vi "RT VI.vi"() -> ()   [LabVIEW 2014]
uses:
  Timer 2013/Control Timer.ctl
  <vilib>/ptbypt/NI_PtbyPt.lvlib
panel:
  out "SDFlag":bool
  in  "Emergency off":bool
  in  "Right":bool
  in  "Center":bool
  in  "Left":bool
  in  "Off":bool
  in  "On":bool
  out "On/Off":bool
  out "BrojacGreska":dbl
  out "Brojac":dbl
  out "Fault":bool
  out "RightLED":bool
  out "CenterLED":bool
  out "LeftLED":bool
  out "Stanje":string
  out "error out":errorcluster
  in  "error in (no error)":errorcluster
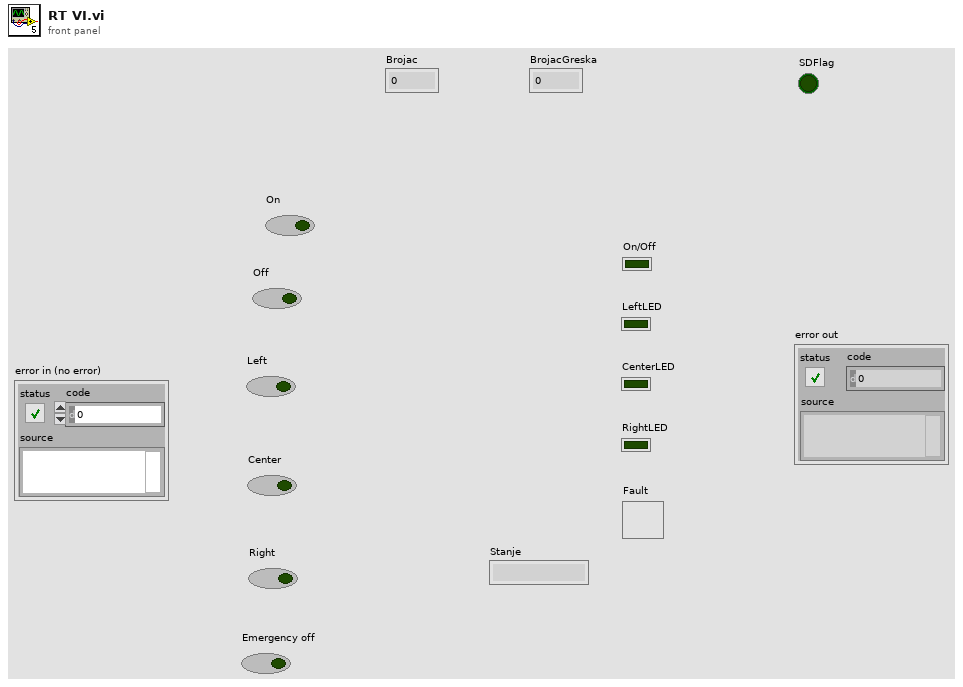
[diagram p1: front panel]
types:
  T1 = typedef "Control Timer.ctl" = enum16{"Timecheck", "Reset"}
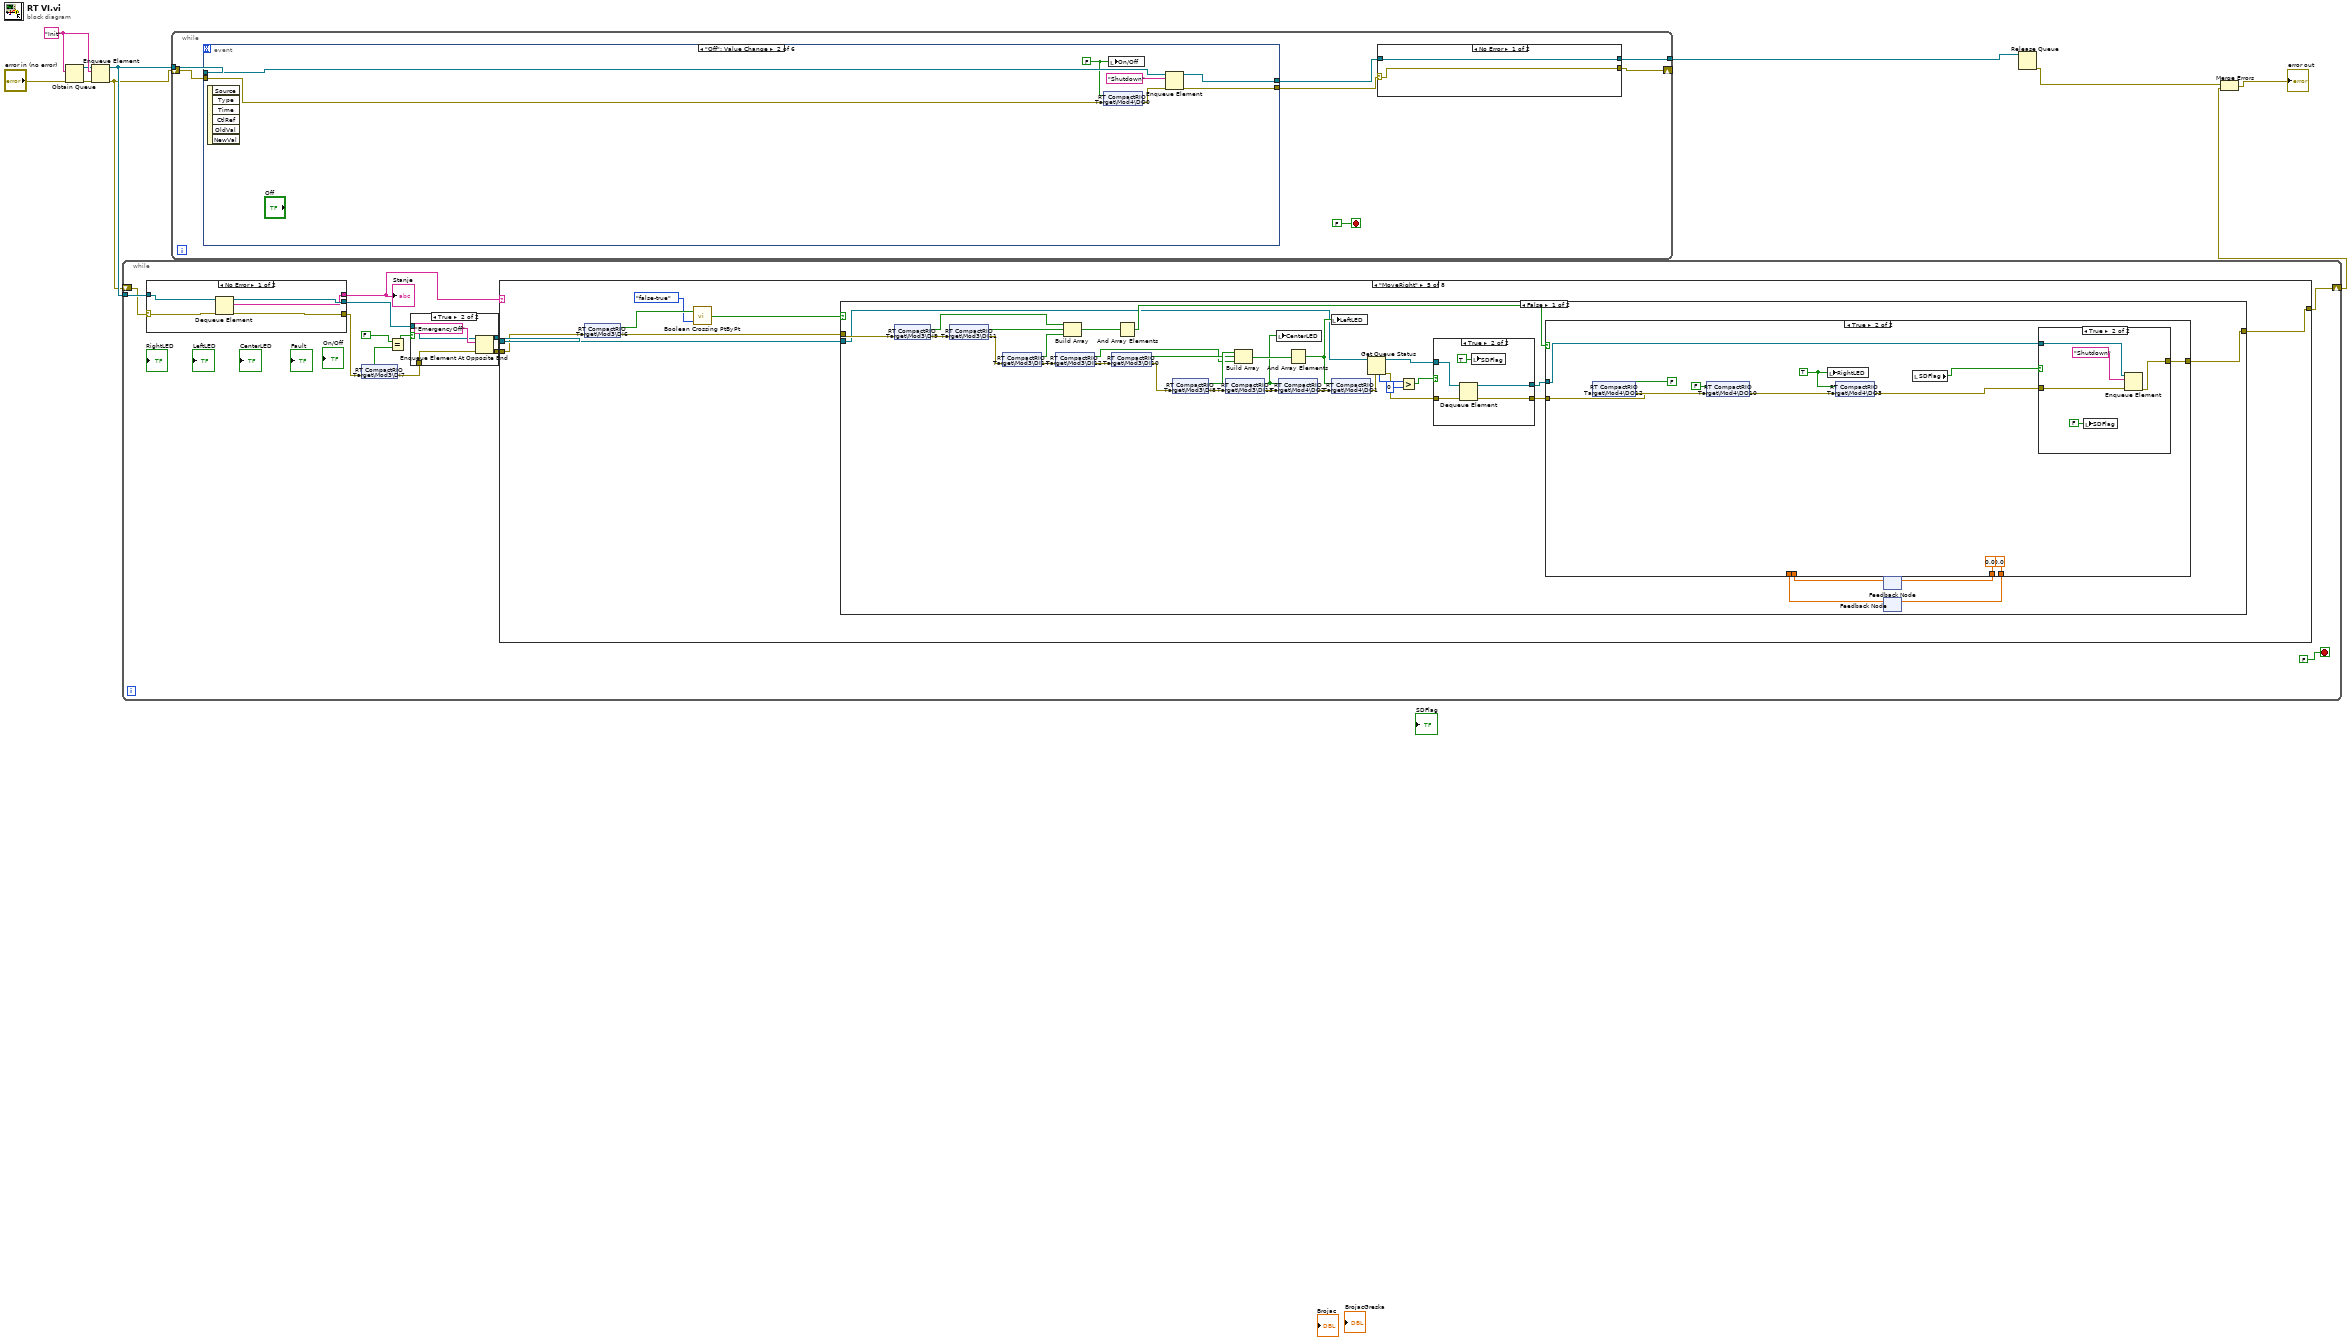
[diagram p0: block diagram]
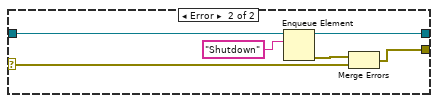
[diagram p2: hidden frame]
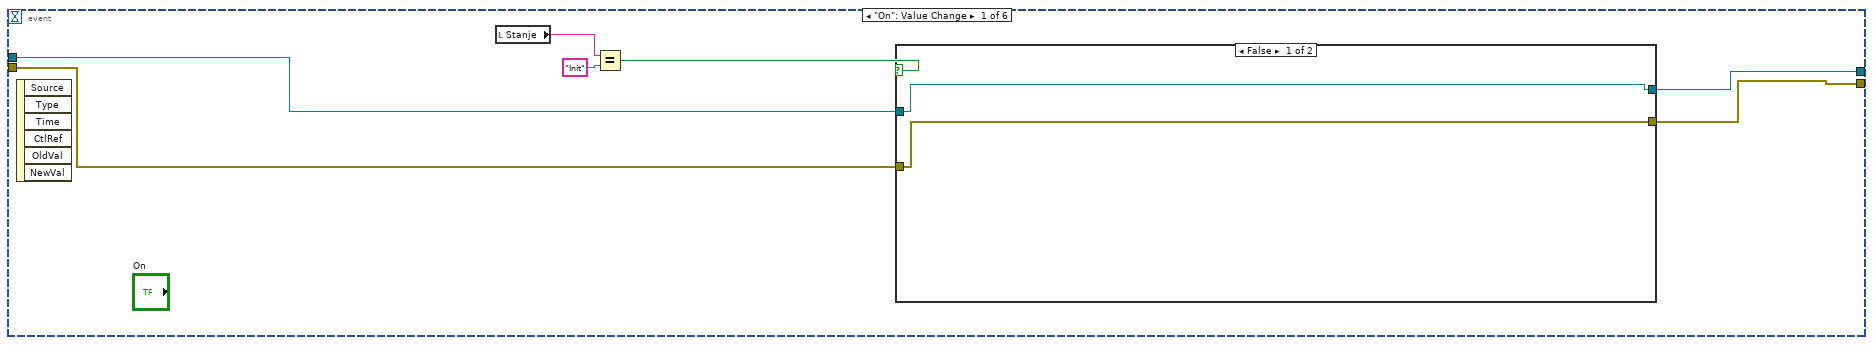
[diagram p3: hidden frame]
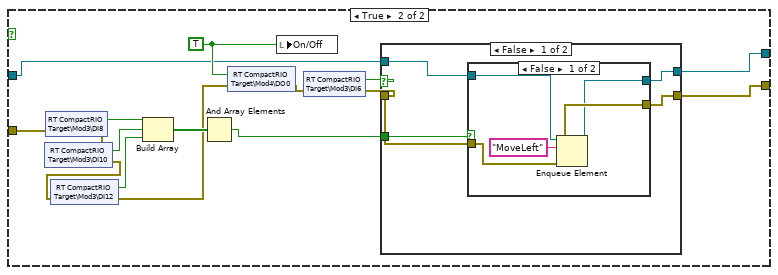
[diagram p4: hidden frame]
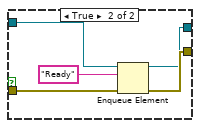
[diagram p5: hidden frame]
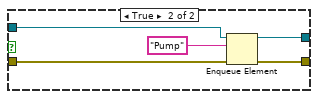
[diagram p6: hidden frame]
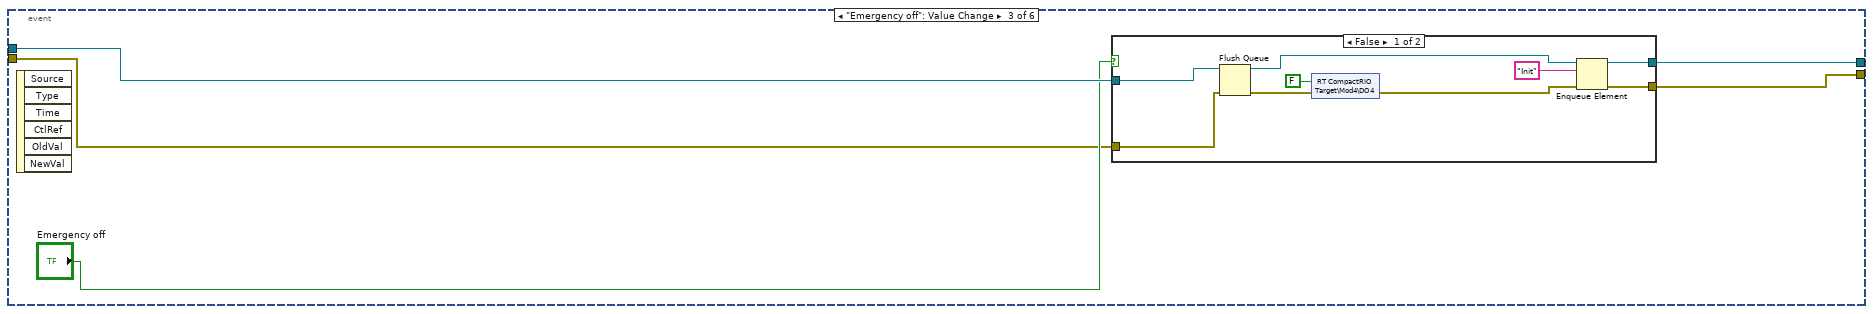
[diagram p7: hidden frame]
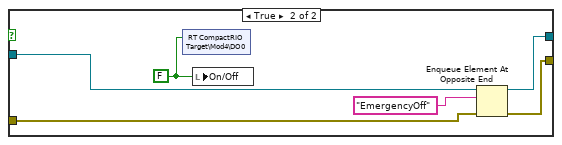
[diagram p8: hidden frame]
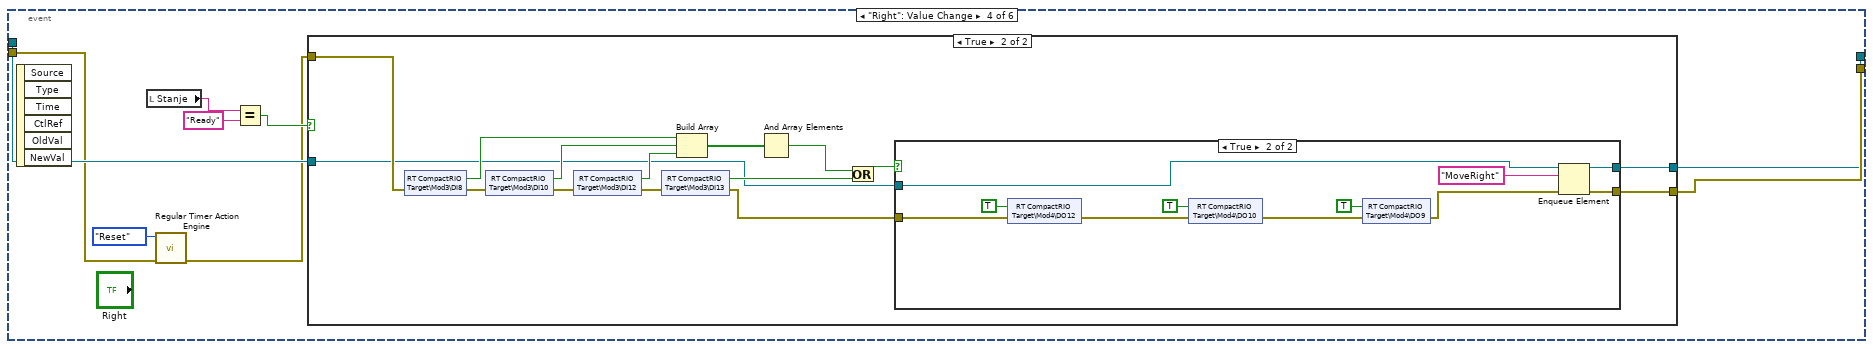
[diagram p9: hidden frame]
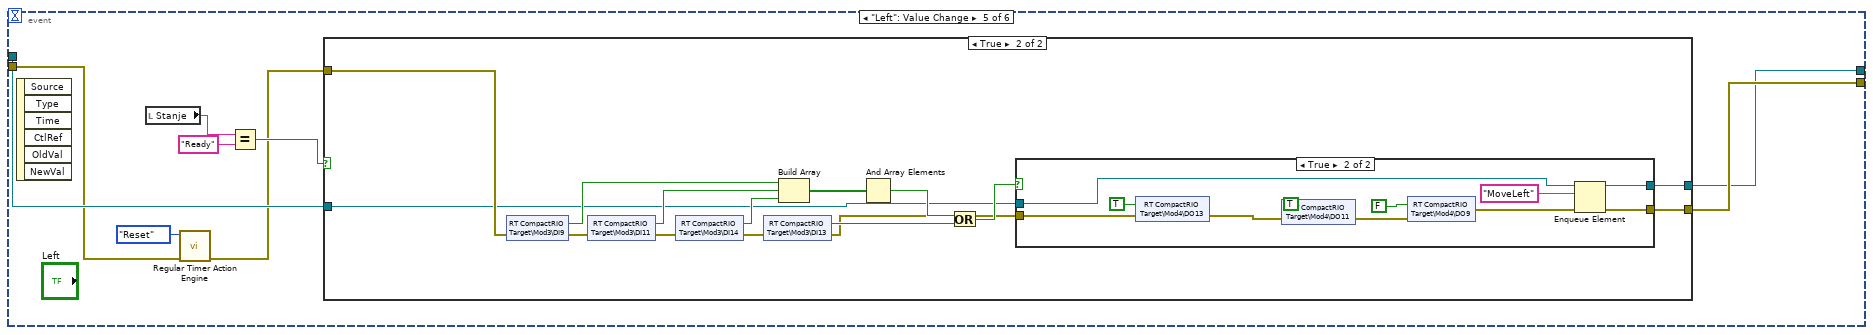
[diagram p12: hidden frame]
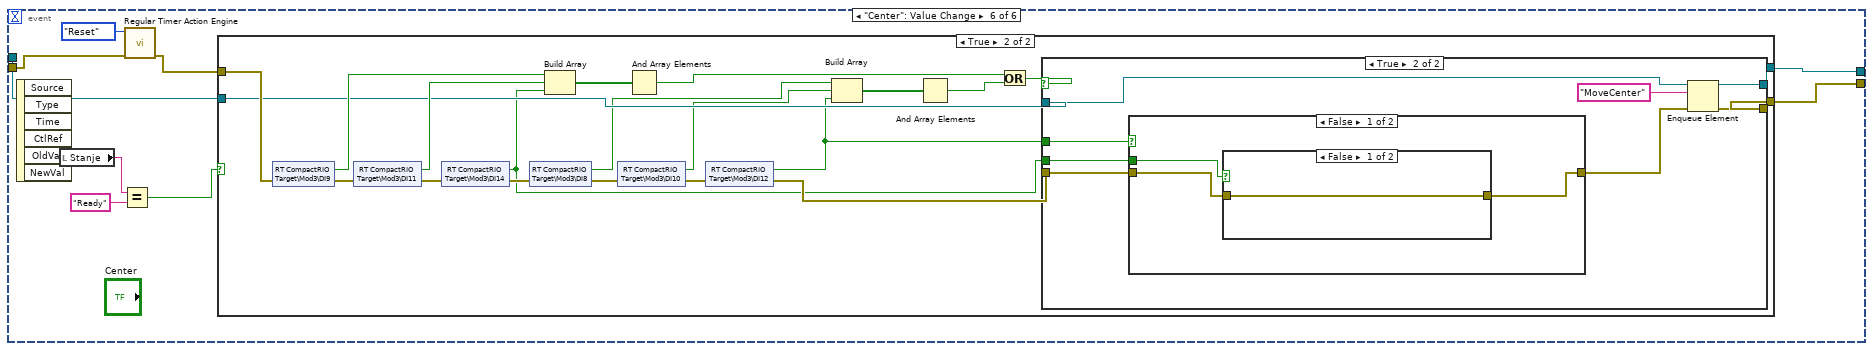
[diagram p15: hidden frame]
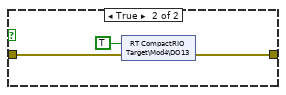
[diagram p18: hidden frame]
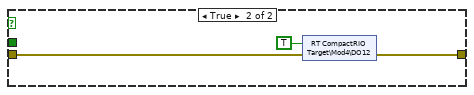
[diagram p19: hidden frame]
diagram:
  w10 = "Init"
  n1 = Obtain Queue(element data type=w10, error in (no error)="error in (no error)") -> (queue out=w8:refnum<queue>, error out=w9:errorcluster)  [unwired: 3 in, 1 out]
  n2 = Enqueue Element(queue=w8, element=w10, error in (no error)=w9) -> (queue out=w7:refnum<queue>, error out=w2:errorcluster)  [unwired: 1 in, 1 out]
  n3 = while {
    tunnel: w7 -> [w23]
    shift-right: [w11] -> w1
    shift-left: w2 -> [w12]
    stop <- FALSE stop-if-true
    n4 = case shown="No Error" w12 {
      selector: w12 -> [w485 w490]
      tunnel: w23 -> [w481 w489]
      tunnel: [w484 w488] -> w21
      tunnel: [w483 w487] -> w15
      tunnel: [w482 w486] -> w22
      frame No Error {
        n5 = Dequeue Element(queue=w481, error in (no error)=w485) -> (queue out=w483:refnum<queue>, element=w482:string, error out=w484:errorcluster)  [unwired: 1 in, 1 out]
      }
      frame Error {
        w486 = "Shutdown" ("element")
        n6 = Enqueue Element(queue=w489, element=w486, error in (no error)=w490) -> (queue out=w487:refnum<queue>, error out=w488:errorcluster)  [unwired: 1 in, 1 out]
      }
    }
    "Stanje" <- w22
    n7 = shared-variable "RT CompactRIO Target\\Mod3\\DI7"(error in=w21) -> (w20:bool, error out=w17:errorcluster)
    n8 = Equal?(x=FALSE, y=w20) -> (x = y?=w18:bool)
    n9 = case shown="True" w18 {
      tunnel: w17 -> [w25 w27]
      tunnel: [w25 w29] -> w16
      tunnel: w15 -> [w24 w26]
      tunnel: [w24 w28] -> w14
      frame False {
      }
      frame True {
        n10 = Enqueue Element At Opposite End(queue=w26, element="EmergencyOff", error in (no error)=w27) -> (queue out=w28:refnum<queue>, error out=w29:errorcluster)  [unwired: 1 in, 1 out]
      }
    }
    n11 = case shown="\"MoveRight\"" w22 {
      selector: w22 -> [_ _ _ _ _ _ _ w474]
      tunnel: [w39 w79 w95 w113 w136 w267 w376 w475] -> w11
      tunnel: w16 -> [w34 w83 w93 w111 w130 w261 w370 w472]
      tunnel: w14 -> [_ w78 w94 w112 w131 w262 w371 w473]
      frame "Init", Default {
        n12 = shared-variable "RT CompactRIO Target\\Mod4\\DO0"(FALSE ("DO0"), error in=w34) -> (error out=w33:errorcluster)
        n13 = shared-variable "RT CompactRIO Target\\Mod3\\DI12"(error in=w33) -> (w69:bool, error out=w67:errorcluster)
        n14 = shared-variable "RT CompactRIO Target\\Mod3\\DI10"(error in=w67) -> (w70:bool, error out=w66:errorcluster)
        n15 = shared-variable "RT CompactRIO Target\\Mod3\\DI8"(error in=w66) -> (w71:bool, error out=w56:errorcluster)
        n16 = Build Array(w71, w70, w69) -> (w68:bool[])
        n17 = And Array Elements(Boolean array=w68) -> (logical AND=w52:bool)
        n18 = local write "LeftLED"(w52) -> ()
        n19 = shared-variable "RT CompactRIO Target\\Mod4\\DO1"(w52, error in=w56) -> (error out=w55:errorcluster)
        n20 = shared-variable "RT CompactRIO Target\\Mod3\\DI14"(error in=w55) -> (w63:bool, error out=w61:errorcluster)
        n21 = shared-variable "RT CompactRIO Target\\Mod3\\DI11"(error in=w61) -> (w64:bool, error out=w60:errorcluster)
        n22 = shared-variable "RT CompactRIO Target\\Mod3\\DI9"(error in=w60) -> (w65:bool, error out=w54:errorcluster)
        n23 = Build Array(w65, w64, w63) -> (w62:bool[])
        n24 = And Array Elements(Boolean array=w62) -> (logical AND=w50:bool)
        n25 = local write "RightLED"(w50) -> ()
        n26 = shared-variable "RT CompactRIO Target\\Mod4\\DO3"(w50, error in=w54) -> (error out=w53:errorcluster)
        n27 = shared-variable "RT CompactRIO Target\\Mod3\\DI13"(error in=w53) -> (w51:bool, error out=w59:errorcluster)
        n28 = local write "Fault"(FALSE) -> ()
        n29 = local write "CenterLED"(w51) -> ()
        n30 = shared-variable "RT CompactRIO Target\\Mod4\\DO2"(w51, error in=w59) -> (error out=w48:errorcluster)
        n31 = shared-variable "RT CompactRIO Target\\Mod4\\DO4"(FALSE ("DO4"), error in=w48) -> (error out=w47:errorcluster)
        n32 = shared-variable "RT CompactRIO Target\\Mod4\\DO13"(FALSE ("DO15"), error in=w47) -> (error out=w32:errorcluster)
        n33 = shared-variable "RT CompactRIO Target\\Mod4\\DO12"(FALSE ("DO14"), error in=w32) -> (error out=w58:errorcluster)
        n34 = shared-variable "RT CompactRIO Target\\Mod4\\DO11"(FALSE ("DO13"), error in=w58) -> (error out=w38:errorcluster)
        n35 = shared-variable "RT CompactRIO Target\\Mod4\\DO8"(FALSE ("DO10"), error in=w38) -> (error out=w37:errorcluster)
        n36 = shared-variable "RT CompactRIO Target\\Mod4\\DO10"(FALSE ("DO12"), error in=w37) -> (error out=w57:errorcluster)
        n37 = shared-variable "RT CompactRIO Target\\Mod4\\DO9"(FALSE ("DO11"), error in=w57) -> (error out=w46:errorcluster)
        n38 = invoke on="On/Off" class="Bool (strict)" method="Reinit To Default"(error in=w46) -> (error out=w36:errorcluster)  [unwired: 2 in, 2 out]
        n39 = invoke on="On" class="Bool (strict)" method="Reinit To Default"(error in=w36) -> (error out=w40:errorcluster)  [unwired: 2 in, 2 out]
        n40 = invoke on="Off" class="Bool (strict)" method="Reinit To Default"(error in=w40) -> (error out=w44:errorcluster)  [unwired: 2 in, 2 out]
        n41 = invoke on="Emergency off" class="Bool (strict)" method="Reinit To Default"(error in=w44) -> (error out=w43:errorcluster)  [unwired: 2 in, 2 out]
        n42 = invoke on="Right" class="Bool (strict)" method="Reinit To Default"(error in=w43) -> (error out=w42:errorcluster)  [unwired: 2 in, 2 out]
        n43 = invoke on="Left" class="Bool (strict)" method="Reinit To Default"(error in=w42) -> (error out=w41:errorcluster)  [unwired: 2 in, 2 out]
        n44 = invoke on="Center" class="Bool (strict)" method="Reinit To Default"(error in=w41) -> (error out=w39:errorcluster)  [unwired: 2 in, 2 out]
      }
      frame "Shutdown" {
        n45 = shared-variable "RT CompactRIO Target\\Mod4\\DO8"(FALSE ("DO8"), error in=w83) -> (error out=w82:errorcluster)
        n46 = shared-variable "RT CompactRIO Target\\Mod4\\DO9"(FALSE ("DO11"), error in=w82) -> (error out=w92:errorcluster)
        n47 = shared-variable "RT CompactRIO Target\\Mod4\\DO10"(FALSE ("DO12"), error in=w92) -> (error out=w84:errorcluster)
        n48 = shared-variable "RT CompactRIO Target\\Mod4\\DO11"(FALSE ("DO13"), error in=w84) -> (error out=w91:errorcluster)
        n49 = shared-variable "RT CompactRIO Target\\Mod4\\DO12"(FALSE ("DO14"), error in=w91) -> (error out=w90:errorcluster)
        n50 = shared-variable "RT CompactRIO Target\\Mod4\\DO13"(FALSE ("DO15"), error in=w90) -> (error out=w80:errorcluster)
        n51 = Enqueue Element(queue=w78, element="Init", error in (no error)=w80) -> (error out=w79:errorcluster)  [unwired: 1 in, 2 out]
      }
      frame "EmergencyOff" {
        w98 = TRUE ("DO4")
        n52 = Enqueue Element At Opposite End(queue=w94, element="EmergencyOff", error in (no error)=w93) -> (error out=w103:errorcluster)  [unwired: 1 in, 2 out]
        n53 = shared-variable "RT CompactRIO Target\\Mod4\\DO12"(FALSE ("DO14"), error in=w103) -> (error out=w100:errorcluster)
        n54 = shared-variable "RT CompactRIO Target\\Mod4\\DO4"(w98, error in=w100) -> (error out=w99:errorcluster)
        n55 = local write "Fault"(w98) -> ()
        n56 = shared-variable "RT CompactRIO Target\\Mod4\\DO13"(FALSE ("DO15"), error in=w99) -> (error out=w102:errorcluster)
        n57 = shared-variable "RT CompactRIO Target\\Mod4\\DO9"(FALSE ("DO11"), error in=w102) -> (error out=w109:errorcluster)
        n58 = shared-variable "RT CompactRIO Target\\Mod4\\DO10"(FALSE ("DO12"), error in=w109) -> (error out=w101:errorcluster)
        n59 = shared-variable "RT CompactRIO Target\\Mod4\\DO11"(FALSE ("DO13"), error in=w101) -> (error out=w97:errorcluster)
        n60 = shared-variable "RT CompactRIO Target\\Mod4\\DO8"(FALSE ("DO8"), error in=w97) -> (error out=w95:errorcluster)
      }
      frame "Pump" {
        n61 = shared-variable "RT CompactRIO Target\\Mod3\\DI6"(error in=w111) -> (w116:bool, error out=w114:errorcluster)
        n62 = call <vilib>:"Boolean Crossing PtByPt.vi"("direction"=enum16{"either", "false-true", "true-false"}."true-false", "input"=w116) -> ("crossing"=w115:bool)  [unwired: 1 in]
        n63 = case shown="True" w115 {
          tunnel: w114 -> [w120 w126]
          tunnel: [w123 w129] -> w113
          tunnel: w112 -> [w118 w124]
          frame False {
            n64 = shared-variable "RT CompactRIO Target\\Mod4\\DO8"(TRUE ("DO10"), error in=w120) -> (error out=w119:errorcluster)
            n65 = Enqueue Element(queue=w118, element="Pump", error in (no error)=w119) -> (error out=w123:errorcluster)  [unwired: 1 in, 2 out]
          }
          frame True {
            n66 = shared-variable "RT CompactRIO Target\\Mod4\\DO8"(FALSE ("DO10"), error in=w126) -> (error out=w125:errorcluster)
            n67 = Enqueue Element(queue=w124, element="Ready", error in (no error)=w125) -> (error out=w129:errorcluster)  [unwired: 1 in, 2 out]
          }
        }
      }
      frame "MoveRight" {
        n68 = shared-variable "RT CompactRIO Target\\Mod3\\DI6"(error in=w130) -> (w134:bool, error out=w135:errorcluster)
        n69 = call <vilib>:"Boolean Crossing PtByPt.vi"("direction"=enum16{"either", "false-true", "true-false"}."false-true", "input"=w134) -> ("crossing"=w132:bool)  [unwired: 1 in]
        n70 = case shown="False" w132 {
          tunnel: w135 -> [w166 w258]
          tunnel: [w163 w259] -> w136
          tunnel: w131 -> [w145 w257]
          frame False {
            n71 = shared-variable "RT CompactRIO Target\\Mod3\\DI9"(error in=w166) -> (w170:bool, error out=w165:errorcluster)
            n72 = shared-variable "RT CompactRIO Target\\Mod3\\DI11"(error in=w165) -> (w169:bool, error out=w164:errorcluster)
            n73 = shared-variable "RT CompactRIO Target\\Mod3\\DI14"(error in=w164) -> (w168:bool, error out=w152:errorcluster)
            n74 = shared-variable "RT CompactRIO Target\\Mod3\\DI12"(error in=w152) -> (w159:bool, error out=w157:errorcluster)
            n75 = Build Array(w170, w169, w168) -> (w167:bool[])
            n76 = shared-variable "RT CompactRIO Target\\Mod3\\DI10"(error in=w157) -> (w160:bool, error out=w156:errorcluster)
            n77 = And Array Elements(Boolean array=w167) -> (logical AND=w162:bool)
            n78 = shared-variable "RT CompactRIO Target\\Mod3\\DI8"(error in=w156) -> (w161:bool, error out=w155:errorcluster)
            n79 = shared-variable "RT CompactRIO Target\\Mod3\\DI13"(error in=w155) -> (w150:bool, error out=w154:errorcluster)
            n80 = Build Array(w161, w160, w159) -> (w158:bool[])
            n81 = local write "CenterLED"(w150) -> ()
            n82 = shared-variable "RT CompactRIO Target\\Mod4\\DO2"(w150, error in=w154) -> (error out=w153:errorcluster)
            n83 = And Array Elements(Boolean array=w158) -> (logical AND=w151:bool)
            n84 = local write "LeftLED"(w151) -> ()
            n85 = shared-variable "RT CompactRIO Target\\Mod4\\DO1"(w151, error in=w153) -> (error out=w144:errorcluster)
            n86 = Get Queue Status(queue=w145, error in (no error)=w144) -> (queue out=w142:refnum<queue>, error out=w143:errorcluster, # elements in queue=w139:i32)  [unwired: 1 in, 5 out]
            n87 = Greater?(x=w139, y=0) -> (0:w137:bool)
            n88 = case shown="True" w137 {
              tunnel: w143 -> [w171 w176]
              tunnel: w142 -> [w172 w175]
              tunnel: [w172 w174] -> w141
              tunnel: [w171 w173] -> w140
              frame False {
              }
              frame True {
                n89 = Dequeue Element(queue=w175, error in (no error)=w176) -> (queue out=w174:refnum<queue>, error out=w173:errorcluster)  [unwired: 1 in, 2 out]
                n90 = local write "SDFlag"(TRUE ("SDFlag")) -> ()
              }
            }
            n91 = feedback #1() -> (w149:dbl)  [unwired: 1 in]
            n92 = feedback #2() -> (w147:dbl)  [unwired: 1 in]
            n93 = case shown="True" w162 {
              tunnel: [w186 w247] -> w163
              tunnel: w149 -> [w183 _]
              tunnel: [w182 0.0] -> w148
              tunnel: w147 -> [w181 _]
              tunnel: [w180 0.0] -> w146
              tunnel: w141 -> [w178 w238]
              tunnel: w140 -> [w179 w237]
              frame False {
                n94 = call "Regular Timer Action Engine.vi"("Enum"=Control_Timer."Timecheck", "Time Target"=0.5, "error in"=w179) -> ("Status"=w192:cluster{"Running":bool, "Done":bool}, "error out"=w189:errorcluster)  [unwired: 6 in]
                n95 = Unbundle By Name(w192) -> ("Done"=w191:bool)  [unwired: 1 out]
                n96 = feedback #3() -> (w190:bool)  [unwired: 1 in]
                n97 = case shown="False" w191 {
                  tunnel: [w200 w219] -> w185
                  tunnel: w190 -> [w200 w218]
                  tunnel: w189 -> [w199 w216]
                  tunnel: [w199 w210] -> w188
                  tunnel: w181 -> [w198 w215]
                  tunnel: [w198 w211] -> w180
                  tunnel: w183 -> [w197 w209]
                  tunnel: [w197 w206] -> w182
                  tunnel: [w196 w205] -> w184
                  tunnel: w178 -> [w196 w201]
                  frame False {
                  }
                  frame True {
                    n98 = Increment(x=w215) -> (x+1=w212:dbl)
                    n99 = Increment(x=w209) -> (x+1=w204:dbl)
                    n100 = local write "Brojac"(w212) -> ()
                    n101 = local write "BrojacGreska"(w204) -> ()
                    n102 = Not(x=w218) -> (.not. x?=w219:bool)
                    n103 = Equal?(x=w204, y=30.0) -> (x = y?=w207:bool)
                    n104 = Equal?(x=4.0, y=w212) -> (x = y?=w214:bool)
                    n105 = call "Regular Timer Action Engine.vi"("Enum"=Control_Timer."Reset", "error in"=w216) -> ("error out"=w203:errorcluster)  [unwired: 7 in, 1 out]
                    n106 = case shown="False" w207 {
                      tunnel: [w222 0.0] -> w206
                      tunnel: w204 -> [w222 _]
                      tunnel: [w220 w226] -> w205
                      tunnel: w203 -> [w221 w225]
                      tunnel: [w221 w224] -> w202
                      tunnel: w201 -> [w220 w223]
                      frame False {
                      }
                      frame True {
                        n107 = Flush Queue(queue=w223, error in (no error)=w225) -> (queue out=w228:refnum<queue>, error out=w229:errorcluster)  [unwired: 1 out]
                        n108 = Enqueue Element At Opposite End(queue=w228, element="EmergencyOff", error in (no error)=w229) -> (queue out=w226:refnum<queue>, error out=w224:errorcluster)  [unwired: 1 in, 1 out]
                      }
                    }
                    n109 = case shown="True" w214 {
                      tunnel: w212 -> [w232 _]
                      tunnel: [w232 0.0] -> w211
                      tunnel: [w231 w233] -> w210
                      tunnel: w202 -> [w231 w233]
                      frame False {
                      }
                      frame True {
                        n110 = shared-variable "RT CompactRIO Target\\Mod4\\DO10"(FALSE ("DO12")) -> ()  [unwired: 1 in, 1 out]
                      }
                    }
                  }
                }
                n111 = feedback-in #3(w185) -> ()
                n112 = local write "RightLED"(w185) -> ()
                n113 = shared-variable "RT CompactRIO Target\\Mod4\\DO3"(w185, error in=w188) -> (error out=w187:errorcluster)
                n114 = Enqueue Element(queue=w184, element="MoveRight", error in (no error)=w187) -> (error out=w186:errorcluster)  [unwired: 1 in, 2 out]
              }
              frame True {
                w241 = TRUE ("DO3")
                n115 = shared-variable "RT CompactRIO Target\\Mod4\\DO12"(FALSE ("DO15"), error in=w237) -> (error out=w244:errorcluster)
                n116 = shared-variable "RT CompactRIO Target\\Mod4\\DO10"(FALSE ("DO13"), error in=w244) -> (error out=w243:errorcluster)
                n117 = local write "RightLED"(w241) -> ()
                n118 = shared-variable "RT CompactRIO Target\\Mod4\\DO3"(w241, error in=w243) -> (error out=w242:errorcluster)
                n119 = local read "SDFlag"() -> (w236:bool)
                n120 = case shown="True" w236 {
                  tunnel: [w250 w256] -> w247
                  tunnel: w242 -> [w249 w252]
                  tunnel: w238 -> [w248 w253]
                  frame False {
                    n121 = Enqueue Element(queue=w248, element="Ready", error in (no error)=w249) -> (error out=w250:errorcluster)  [unwired: 1 in, 2 out]
                  }
                  frame True {
                    n122 = local write "SDFlag"(FALSE ("SDFlag")) -> ()
                    n123 = Enqueue Element(queue=w253, element="Shutdown", error in (no error)=w252) -> (error out=w256:errorcluster)  [unwired: 1 in, 2 out]
                  }
                }
              }
            }
            n124 = feedback-in #1(w148) -> ()
            n125 = feedback-in #2(w146) -> ()
          }
          frame True {
            n126 = Enqueue Element(queue=w257, element="Pump", error in (no error)=w258) -> (error out=w259:errorcluster)  [unwired: 1 in, 2 out]
          }
        }
      }
      frame "MoveLeft" {
        n127 = shared-variable "RT CompactRIO Target\\Mod3\\DI6"(error in=w261) -> (w266:bool, error out=w264:errorcluster)
        n128 = call <vilib>:"Boolean Crossing PtByPt.vi"("direction"=enum16{"either", "false-true", "true-false"}."false-true", "input"=w266) -> ("crossing"=w263:bool)  [unwired: 1 in]
        n129 = case shown="False" w263 {
          tunnel: w264 -> [w289 w366]
          tunnel: [w286 w368] -> w267
          tunnel: w262 -> [w272 w367]
          frame False {
            n130 = shared-variable "RT CompactRIO Target\\Mod3\\DI8"(error in=w289) -> (w294:bool, error out=w288:errorcluster)
            n131 = shared-variable "RT CompactRIO Target\\Mod3\\DI10"(error in=w288) -> (w293:bool, error out=w287:errorcluster)
            n132 = shared-variable "RT CompactRIO Target\\Mod3\\DI12"(error in=w287) -> (w292:bool, error out=w281:errorcluster)
            n133 = shared-variable "RT CompactRIO Target\\Mod3\\DI14"(error in=w281) -> (w283:bool, error out=w280:errorcluster)
            n134 = Build Array(w294, w293, w292) -> (w291:bool[])
            n135 = shared-variable "RT CompactRIO Target\\Mod3\\DI11"(error in=w280) -> (w284:bool, error out=w279:errorcluster)
            n136 = And Array Elements(Boolean array=w291) -> (logical AND=w290:bool)
            n137 = shared-variable "RT CompactRIO Target\\Mod3\\DI9"(error in=w279) -> (w285:bool, error out=w278:errorcluster)
            n138 = shared-variable "RT CompactRIO Target\\Mod3\\DI13"(error in=w278) -> (w273:bool, error out=w277:errorcluster)
            n139 = Build Array(w285, w284, w283) -> (w282:bool[])
            n140 = local write "CenterLED"(w273) -> ()
            n141 = shared-variable "RT CompactRIO Target\\Mod4\\DO2"(w273, error in=w277) -> (error out=w276:errorcluster)
            n142 = And Array Elements(Boolean array=w282) -> (logical AND=w274:bool)
            n143 = local write "RightLED"(w274) -> ()
            n144 = shared-variable "RT CompactRIO Target\\Mod4\\DO3"(w274, error in=w276) -> (error out=w275:errorcluster)
            n145 = feedback #4() -> (w271:dbl)  [unwired: 1 in]
            n146 = feedback #5() -> (w269:dbl)  [unwired: 1 in]
            n147 = case shown="False" w290 {
              tunnel: w275 -> [w299 w360]
              tunnel: [w312 w364] -> w286
              tunnel: w272 -> [w302 w356]
              tunnel: w271 -> [w298 _]
              tunnel: [w297 0.0] -> w270
              tunnel: w269 -> [w296 _]
              tunnel: [w295 0.0] -> w268
              frame False {
                n148 = call "Regular Timer Action Engine.vi"("Enum"=Control_Timer."Timecheck", "Time Target"=0.5, "error in"=w299) -> ("Status"=w308:cluster{"Running":bool, "Done":bool}, "error out"=w305:errorcluster)  [unwired: 6 in]
                n149 = Unbundle By Name(w308) -> ("Done"=w307:bool)  [unwired: 1 out]
                n150 = feedback #6() -> (w306:bool)  [unwired: 1 in]
                n151 = case shown="True" w307 {
                  tunnel: [w317 w336] -> w303
                  tunnel: w306 -> [w317 w335]
                  tunnel: w305 -> [w316 w324]
                  tunnel: [w316 w333] -> w300
                  tunnel: [w315 w329] -> w295
                  tunnel: w296 -> [w315 w332]
                  tunnel: w298 -> [w314 w320]
                  tunnel: w302 -> [w313 w326]
                  tunnel: [w313 w325] -> w301
                  tunnel: [w314 w321] -> w297
                  frame False {
                  }
                  frame True {
                    n152 = Increment(x=w332) -> (x+1=w319:dbl)
                    n153 = local write "Brojac"(w319) -> ()
                    n154 = Increment(x=w320) -> (x+1=w318:dbl)
                    n155 = local write "BrojacGreska"(w318) -> ()
                    n156 = Equal?(x=w318, y=30.0) -> (x = y?=w327:bool)
                    n157 = Equal?(x=w319, y=4.0) -> (x = y?=w330:bool)
                    n158 = Not(x=w335) -> (.not. x?=w336:bool)
                    n159 = case shown="True" w330 {
                      tunnel: w319 -> [w349 _]
                      tunnel: [w349 0.0] -> w329
                      tunnel: w324 -> [w348 w351]
                      tunnel: [w348 w350] -> w323
                      frame False {
                      }
                      frame True {
                        n160 = shared-variable "RT CompactRIO Target\\Mod4\\DO11"(FALSE ("DO13"), error in=w351) -> (error out=w350:errorcluster)
                      }
                    }
                    n161 = case shown="True" w327 {
                      tunnel: w318 -> [w339 _]
                      tunnel: [w339 0.0] -> w321
                      tunnel: w326 -> [w338 w346]
                      tunnel: [w338 w344] -> w325
                      tunnel: w323 -> [w337 w343]
                      tunnel: [w337 w341] -> w322
                      frame False {
                      }
                      frame True {
                        n162 = Flush Queue(queue=w346, error in (no error)=w343) -> (queue out=w345:refnum<queue>, error out=w342:errorcluster)  [unwired: 1 out]
                        n163 = Enqueue Element At Opposite End(queue=w345, element="EmergencyOff", error in (no error)=w342) -> (queue out=w344:refnum<queue>, error out=w341:errorcluster)  [unwired: 1 in, 1 out]
                      }
                    }
                    n164 = call "Regular Timer Action Engine.vi"("Enum"=Control_Timer."Reset", "error in"=w322) -> ("error out"=w333:errorcluster)  [unwired: 7 in, 1 out]
                  }
                }
                n165 = feedback-in #6(w303) -> ()
                n166 = local write "LeftLED"(w303) -> ()
                n167 = shared-variable "RT CompactRIO Target\\Mod4\\DO1"(w303, error in=w300) -> (error out=w304:errorcluster)
                n168 = Enqueue Element(queue=w301, element="MoveLeft", error in (no error)=w304) -> (error out=w312:errorcluster)  [unwired: 1 in, 2 out]
              }
              frame True {
                w358 = TRUE ("DO1")
                # "flushovali queue"
                n169 = local write "LeftLED"(w358) -> ()
                n170 = shared-variable "RT CompactRIO Target\\Mod4\\DO1"(w358, error in=w360) -> (error out=w359:errorcluster)
                n171 = shared-variable "RT CompactRIO Target\\Mod4\\DO13"(FALSE ("DO15"), error in=w359) -> (error out=w361:errorcluster)
                n172 = shared-variable "RT CompactRIO Target\\Mod4\\DO11"(FALSE ("DO13"), error in=w361) -> (error out=w357:errorcluster)
                n173 = Enqueue Element(queue=w356, element="Ready", error in (no error)=w357) -> (error out=w364:errorcluster)  [unwired: 1 in, 2 out]
              }
            }
            n174 = feedback-in #4(w270) -> ()
            n175 = feedback-in #5(w268) -> ()
          }
          frame True {
            n176 = Enqueue Element(queue=w367, element="Pump", error in (no error)=w366) -> (error out=w368:errorcluster)  [unwired: 1 in, 2 out]
          }
        }
      }
      frame "MoveCenter" {
        n177 = shared-variable "RT CompactRIO Target\\Mod3\\DI6"(error in=w370) -> (w375:bool, error out=w372:errorcluster)
        n178 = call <vilib>:"Boolean Crossing PtByPt.vi"("direction"=enum16{"either", "false-true", "true-false"}."false-true", "input"=w375) -> ("crossing"=w373:bool)  [unwired: 1 in]
        n179 = case shown="False" w373 {
          tunnel: [w401 w459] -> w376
          tunnel: w372 -> [w386 w458]
          tunnel: w371 -> [w379 w457]
          frame False {
            n180 = shared-variable "RT CompactRIO Target\\Mod3\\DI12"(error in=w386) -> (w396:bool, error out=w394:errorcluster)
            n181 = shared-variable "RT CompactRIO Target\\Mod3\\DI10"(error in=w394) -> (w397:bool, error out=w393:errorcluster)
            n182 = shared-variable "RT CompactRIO Target\\Mod3\\DI8"(error in=w393) -> (w398:bool, error out=w385:errorcluster)
            n183 = shared-variable "RT CompactRIO Target\\Mod3\\DI14"(error in=w385) -> (w390:bool, error out=w388:errorcluster)
            n184 = Build Array(w398, w397, w396) -> (w395:bool[])
            n185 = shared-variable "RT CompactRIO Target\\Mod3\\DI11"(error in=w388) -> (w391:bool, error out=w387:errorcluster)
            n186 = And Array Elements(Boolean array=w395) -> (logical AND=w380:bool)
            n187 = local write "LeftLED"(w380) -> ()
            n188 = shared-variable "RT CompactRIO Target\\Mod3\\DI9"(error in=w387) -> (w392:bool, error out=w384:errorcluster)
            n189 = shared-variable "RT CompactRIO Target\\Mod4\\DO1"(w380, error in=w384) -> (error out=w383:errorcluster)
            n190 = Build Array(w392, w391, w390) -> (w389:bool[])
            n191 = And Array Elements(Boolean array=w389) -> (logical AND=w381:bool)
            n192 = local write "RightLED"(w381) -> ()
            n193 = shared-variable "RT CompactRIO Target\\Mod4\\DO3"(w381, error in=w383) -> (error out=w382:errorcluster)
            n194 = shared-variable "RT CompactRIO Target\\Mod3\\DI13"(error in=w382) -> (w400:bool, error out=w399:errorcluster)
            n195 = feedback #7() -> (w378:dbl)  [unwired: 1 in]
            n196 = case shown="False" w400 {
              tunnel: [w409 w455] -> w401
              tunnel: w399 -> [w410 w453]
              tunnel: w379 -> [w405 w448]
              tunnel: [w403 0.0] -> w377
              tunnel: w378 -> [w402 _]
              frame False {
                n197 = call "Regular Timer Action Engine.vi"("Enum"=Control_Timer."Timecheck", "Time Target"=0.5, "error in"=w410) -> ("Status"=w414:cluster{"Running":bool, "Done":bool}, "error out"=w411:errorcluster)  [unwired: 6 in]
                n198 = Unbundle By Name(w414) -> ("Done"=w413:bool)  [unwired: 1 out]
                n199 = feedback #8() -> (w412:bool)  [unwired: 1 in]
                n200 = case shown="False" w413 {
                  tunnel: [w421 w434] -> w406
                  tunnel: w412 -> [w421 w433]
                  tunnel: w411 -> [w420 w425]
                  tunnel: [w420 w431] -> w408
                  tunnel: w405 -> [w419 w427]
                  tunnel: [w419 w426] -> w404
                  tunnel: [w418 w423] -> w403
                  tunnel: w402 -> [w418 w422]
                  frame False {
                  }
                  frame True {
                    n201 = Increment(x=w422) -> (x+1=w428:dbl)
                    n202 = local write "BrojacGreska"(w428) -> ()
                    n203 = Equal?(x=w428, y=30.0) -> (x = y?=w429:bool)
                    n204 = case shown="True" w429 {
                      tunnel: [w437 0.0] -> w423
                      tunnel: w428 -> [w437 _]
                      tunnel: w427 -> [w435 w443]
                      tunnel: [w435 w441] -> w426
                      tunnel: w425 -> [w436 w440]
                      tunnel: [w436 w438] -> w424
                      frame False {
                      }
                      frame True {
                        n205 = Flush Queue(queue=w443, error in (no error)=w440) -> (queue out=w442:refnum<queue>, error out=w439:errorcluster)  [unwired: 1 out]
                        n206 = Enqueue Element At Opposite End(queue=w442, element="EmergencyOff", error in (no error)=w439) -> (queue out=w441:refnum<queue>, error out=w438:errorcluster)  [unwired: 1 in, 1 out]
                      }
                    }
                    n207 = Not(x=w433) -> (.not. x?=w434:bool)
                    n208 = call "Regular Timer Action Engine.vi"("Enum"=Control_Timer."Reset", "error in"=w424) -> ("error out"=w431:errorcluster)  [unwired: 7 in, 1 out]
                  }
                }
                n209 = feedback-in #8(w406) -> ()
                n210 = local write "CenterLED"(w406) -> ()
                n211 = shared-variable "RT CompactRIO Target\\Mod4\\DO2"(w406, error in=w408) -> (error out=w407:errorcluster)
                n212 = Enqueue Element(queue=w404, element="MoveCenter", error in (no error)=w407) -> (error out=w409:errorcluster)  [unwired: 1 in, 2 out]
              }
              frame True {
                w449 = TRUE ("DO2")
                n213 = shared-variable "RT CompactRIO Target\\Mod4\\DO13"(FALSE ("DO15"), error in=w453) -> (error out=w452:errorcluster)
                n214 = shared-variable "RT CompactRIO Target\\Mod4\\DO12"(FALSE ("DO14"), error in=w452) -> (error out=w451:errorcluster)
                n215 = local write "CenterLED"(w449) -> ()
                n216 = shared-variable "RT CompactRIO Target\\Mod4\\DO2"(w449, error in=w451) -> (error out=w450:errorcluster)
                n217 = Enqueue Element(queue=w448, element="Ready", error in (no error)=w450) -> (error out=w455:errorcluster)  [unwired: 1 in, 2 out]
              }
            }
            n218 = feedback-in #7(w377) -> ()
          }
          frame True {
            n219 = Enqueue Element(queue=w457, element="Pump", error in (no error)=w458) -> (error out=w459:errorcluster)  [unwired: 1 in, 2 out]
          }
        }
      }
      frame "Ready" {
        n220 = Preview Queue Element(queue=w473, error in (no error)=w472) -> (queue out=w471:refnum<queue>, element=w468:string, error out=w470:errorcluster)  [unwired: 1 in, 1 out]
        n221 = Equal?(x=w468, y="MoveRight") -> (x = y?=w465:bool)
        n222 = Equal?(x=w468, y="MoveLeft") -> (x = y?=w464:bool)
        n223 = Equal?(x=w468, y="MoveCenter") -> (x = y?=w462:bool)
        n224 = Or(x=w465, y=w464) -> (x .or. y?=w463:bool)
        n225 = Or(x=w463, y=w462) -> (x .or. y?=w461:bool)
        n226 = case shown="False" w461 {
          tunnel: [w479 w480] -> w475
          tunnel: w474 -> [w478 _]
          tunnel: w471 -> [w477 _]
          tunnel: w470 -> [w476 w480]
          frame False {
            n227 = Enqueue Element(queue=w477, element=w478, error in (no error)=w476) -> (error out=w479:errorcluster)  [unwired: 1 in, 2 out]
          }
          frame True {
          }
        }
      }
    }
  }
  n228 = while {
    tunnel: w7 -> [w497]
    tunnel: [w494] -> w5
    shift-right: [w492] -> _
    shift-left: w2 -> [w491]
    stop <- FALSE stop-if-true
    n229 = event shown="[1] \"Off\": Value Change" {
      selector: _ -> [_ _ _ _ _ _]
      dyn-events: _ -> [_ _ _ _ _ _]
      timeout: _ -> [_ _ _ _ _ _]
      tunnel: w497 -> [w507 w556 w562 w584 w623 w662]
      tunnel: [w512 w555 w561 w586 w625 w664] -> w496
      tunnel: [w511 w554 w560 w585 w624 w663] -> w495
      tunnel: w491 -> [w506 w551 w558 w578 w617 w656]
      event "On": Value Change {
        n230 = event-data() -> ()  [unwired: 1 in, 6 out]
        n231 = local read "Stanje"() -> (w508:string)
        n232 = Equal?(x=w508, y="Init") -> (x = y?=w509:bool)
        n233 = case shown="False" w509 {
          tunnel: [w513 w530] -> w512
          tunnel: [w514 w529] -> w511
          tunnel: w507 -> [w514 w516]
          tunnel: w506 -> [w513 w515]
          frame False {
          }
          frame True {
            w517 = TRUE
            n234 = shared-variable "RT CompactRIO Target\\Mod3\\DI8"(error in=w515) -> (w523:bool, error out=w520:errorcluster)
            n235 = shared-variable "RT CompactRIO Target\\Mod3\\DI10"(error in=w520) -> (w524:bool, error out=w519:errorcluster)
            n236 = shared-variable "RT CompactRIO Target\\Mod3\\DI12"(error in=w519) -> (w525:bool, error out=w518:errorcluster)
            n237 = Build Array(w523, w524, w525) -> (w522:bool[])
            n238 = And Array Elements(Boolean array=w522) -> (logical AND=w521:bool)
            n239 = shared-variable "RT CompactRIO Target\\Mod4\\DO0"(w517, error in=w518) -> (error out=w526:errorcluster)
            n240 = local write "On/Off"(w517) -> ()
            n241 = shared-variable "RT CompactRIO Target\\Mod3\\DI6"(error in=w526) -> (w528:bool, error out=w527:errorcluster)
            n242 = case shown="False" w528 {
              tunnel: [w535 w549] -> w530
              tunnel: [w534 w548] -> w529
              tunnel: w527 -> [w533 w547]
              tunnel: w521 -> [w532 _]
              tunnel: w516 -> [w531 w546]
              frame False {
                n243 = case shown="False" w532 {
                  tunnel: [w539 w545] -> w535
                  tunnel: [w538 w543] -> w534
                  tunnel: w533 -> [w540 w542]
                  tunnel: w531 -> [w536 w541]
                  frame False {
                    n244 = Enqueue Element(queue=w536, element="MoveLeft", error in (no error)=w540) -> (queue out=w538:refnum<queue>, error out=w539:errorcluster)  [unwired: 1 in, 1 out]
                  }
                  frame True {
                    n245 = Enqueue Element(queue=w541, element="Ready", error in (no error)=w542) -> (queue out=w543:refnum<queue>, error out=w545:errorcluster)  [unwired: 1 in, 1 out]
                  }
                }
              }
              frame True {
                n246 = Enqueue Element(queue=w546, element="Pump", error in (no error)=w547) -> (queue out=w548:refnum<queue>, error out=w549:errorcluster)  [unwired: 1 in, 1 out]
              }
            }
          }
        }
      }
      event "Off": Value Change {
        w552 = FALSE
        n247 = event-data() -> ()  [unwired: 1 in, 6 out]
        n248 = shared-variable "RT CompactRIO Target\\Mod4\\DO0"(w552, error in=w551) -> (error out=w553:errorcluster)
        n249 = local write "On/Off"(w552) -> ()
        n250 = Enqueue Element(queue=w556, element="Shutdown", error in (no error)=w553) -> (queue out=w554:refnum<queue>, error out=w555:errorcluster)  [unwired: 1 in, 1 out]
      }
      event "Emergency off": Value Change {
        n251 = event-data() -> ()  [unwired: 1 in, 6 out]
        n252 = case shown="False" "Emergency off" {
          tunnel: w562 -> [w571 w576]
          tunnel: [w570 w575] -> w561
          tunnel: [w569 w574] -> w560
          tunnel: w558 -> [w563 w572]
          frame False {
            n253 = Flush Queue(queue=w571, error in (no error)=w563) -> (queue out=w568:refnum<queue>, error out=w565:errorcluster)  [unwired: 1 out]
            n254 = shared-variable "RT CompactRIO Target\\Mod4\\DO4"(FALSE ("DO4"), error in=w565) -> (error out=w564:errorcluster)
            n255 = Enqueue Element(queue=w568, element="Init", error in (no error)=w564) -> (queue out=w569:refnum<queue>, error out=w570:errorcluster)  [unwired: 1 in, 1 out]
          }
          frame True {
            w573 = FALSE
            n256 = shared-variable "RT CompactRIO Target\\Mod4\\DO0"(w573) -> ()  [unwired: 1 in, 1 out]
            n257 = local write "On/Off"(w573) -> ()
            n258 = Enqueue Element At Opposite End(queue=w576, element="EmergencyOff", error in (no error)=w572) -> (queue out=w574:refnum<queue>, error out=w575:errorcluster)  [unwired: 1 in, 1 out]
          }
        }
      }
      event "Right": Value Change {
        n259 = event-data() -> ()  [unwired: 1 in, 6 out]
        n260 = local read "Stanje"() -> (w583:string)
        n261 = call "Regular Timer Action Engine.vi"("Enum"=Control_Timer."Reset", "error in"=w578) -> ("error out"=w579:errorcluster)  [unwired: 7 in, 1 out]
        n262 = Equal?(x=w583, y="Ready") -> (x = y?=w581:bool)
        n263 = case shown="True" w581 {
          tunnel: w579 -> [w588 w596]
          tunnel: [w588 w591] -> w586
          tunnel: [w587 w590] -> w585
          tunnel: w584 -> [w587 w589]
          frame False {
          }
          frame True {
            n264 = shared-variable "RT CompactRIO Target\\Mod3\\DI8"(error in=w596) -> (w601:bool, error out=w595:errorcluster)
            n265 = shared-variable "RT CompactRIO Target\\Mod3\\DI10"(error in=w595) -> (w602:bool, error out=w594:errorcluster)
            n266 = shared-variable "RT CompactRIO Target\\Mod3\\DI12"(error in=w594) -> (w603:bool, error out=w593:errorcluster)
            n267 = shared-variable "RT CompactRIO Target\\Mod3\\DI13"(error in=w593) -> (w599:bool, error out=w592:errorcluster)
            n268 = Build Array(w601, w602, w603) -> (w600:bool[])
            n269 = And Array Elements(Boolean array=w600) -> (logical AND=w597:bool)
            n270 = Or(x=w597, y=w599) -> (x .or. y?=w598:bool)
            n271 = case shown="True" w598 {
              tunnel: w592 -> [w605 w610]
              tunnel: [w605 w615] -> w591
              tunnel: [w604 w614] -> w590
              tunnel: w589 -> [w604 w606]
              frame False {
              }
              frame True {
                n272 = shared-variable "RT CompactRIO Target\\Mod4\\DO12"(TRUE ("DO15"), error in=w610) -> (error out=w609:errorcluster)
                n273 = shared-variable "RT CompactRIO Target\\Mod4\\DO10"(TRUE ("DO13"), error in=w609) -> (error out=w608:errorcluster)
                n274 = shared-variable "RT CompactRIO Target\\Mod4\\DO9"(TRUE ("DO11"), error in=w608) -> (error out=w607:errorcluster)
                n275 = Enqueue Element(queue=w606, element="MoveRight", error in (no error)=w607) -> (queue out=w614:refnum<queue>, error out=w615:errorcluster)  [unwired: 1 in, 1 out]
              }
            }
          }
        }
      }
      event "Left": Value Change {
        n276 = event-data() -> ()  [unwired: 1 in, 6 out]
        n277 = local read "Stanje"() -> (w622:string)
        n278 = call "Regular Timer Action Engine.vi"("Enum"=Control_Timer."Reset", "error in"=w617) -> ("error out"=w618:errorcluster)  [unwired: 7 in, 1 out]
        n279 = Equal?(x=w622, y="Ready") -> (x = y?=w620:bool)
        n280 = case shown="True" w620 {
          tunnel: w618 -> [w627 w635]
          tunnel: [w627 w630] -> w625
          tunnel: [w626 w629] -> w624
          tunnel: w623 -> [w626 w628]
          frame False {
          }
          frame True {
            n281 = shared-variable "RT CompactRIO Target\\Mod3\\DI9"(error in=w635) -> (w640:bool, error out=w634:errorcluster)
            n282 = shared-variable "RT CompactRIO Target\\Mod3\\DI11"(error in=w634) -> (w641:bool, error out=w633:errorcluster)
            n283 = shared-variable "RT CompactRIO Target\\Mod3\\DI14"(error in=w633) -> (w642:bool, error out=w632:errorcluster)
            n284 = shared-variable "RT CompactRIO Target\\Mod3\\DI13"(error in=w632) -> (w638:bool, error out=w631:errorcluster)
            n285 = Build Array(w640, w641, w642) -> (w639:bool[])
            n286 = And Array Elements(Boolean array=w639) -> (logical AND=w636:bool)
            n287 = Or(x=w636, y=w638) -> (x .or. y?=w637:bool)
            n288 = case shown="True" w637 {
              tunnel: w631 -> [w644 w649]
              tunnel: [w644 w654] -> w630
              tunnel: [w643 w652] -> w629
              tunnel: w628 -> [w643 w653]
              frame False {
              }
              frame True {
                n289 = shared-variable "RT CompactRIO Target\\Mod4\\DO13"(TRUE ("DO15"), error in=w649) -> (error out=w648:errorcluster)
                n290 = shared-variable "RT CompactRIO Target\\Mod4\\DO11"(TRUE ("DO13"), error in=w648) -> (error out=w647:errorcluster)
                n291 = shared-variable "RT CompactRIO Target\\Mod4\\DO9"(FALSE ("DO9"), error in=w647) -> (error out=w646:errorcluster)
                n292 = Enqueue Element(queue=w653, element="MoveLeft", error in (no error)=w646) -> (queue out=w652:refnum<queue>, error out=w654:errorcluster)  [unwired: 1 in, 1 out]
              }
            }
          }
        }
      }
      event "Center": Value Change {
        n293 = event-data() -> ()  [unwired: 1 in, 6 out]
        n294 = local read "Stanje"() -> (w659:string)
        n295 = Equal?(x=w659, y="Ready") -> (x = y?=w660:bool)
        n296 = call "Regular Timer Action Engine.vi"("Enum"=Control_Timer."Reset", "error in"=w656) -> ("error out"=w658:errorcluster)  [unwired: 7 in, 1 out]
        n297 = case shown="True" w660 {
          tunnel: w658 -> [w666 w682]
          tunnel: [w666 w679] -> w664
          tunnel: [w665 w678] -> w663
          tunnel: w662 -> [w665 w677]
          frame False {
          }
          frame True {
            n298 = shared-variable "RT CompactRIO Target\\Mod3\\DI9"(error in=w682) -> (w686:bool, error out=w681:errorcluster)
            n299 = shared-variable "RT CompactRIO Target\\Mod3\\DI11"(error in=w681) -> (w687:bool, error out=w680:errorcluster)
            n300 = shared-variable "RT CompactRIO Target\\Mod3\\DI14"(error in=w680) -> (w667:bool, error out=w673:errorcluster)
            n301 = shared-variable "RT CompactRIO Target\\Mod3\\DI8"(error in=w673) -> (w675:bool, error out=w672:errorcluster)
            n302 = Build Array(w686, w687, w667) -> (w685:bool[])
            n303 = shared-variable "RT CompactRIO Target\\Mod3\\DI10"(error in=w672) -> (w676:bool, error out=w671:errorcluster)
            n304 = And Array Elements(Boolean array=w685) -> (logical AND=w683:bool)
            n305 = shared-variable "RT CompactRIO Target\\Mod3\\DI12"(error in=w671) -> (w668:bool, error out=w670:errorcluster)
            n306 = Build Array(w675, w676, w668) -> (w674:bool[])
            n307 = And Array Elements(Boolean array=w674) -> (logical AND=w669:bool)
            n308 = Or(x=w683, y=w669) -> (x .or. y?=w684:bool)
            n309 = case shown="True" w684 {
              tunnel: w670 -> [w689 w691]
              tunnel: [w689 w696] -> w679
              tunnel: [w688 w694] -> w678
              tunnel: w677 -> [w688 w695]
              tunnel: w668 -> [_ w693]
              tunnel: w667 -> [_ w692]
              frame False {
              }
              frame True {
                n310 = case shown="False" w693 {
                  tunnel: w692 -> [w700 _]
                  tunnel: w691 -> [w699 w706]
                  tunnel: [w698 w705] -> w690
                  frame False {
                    n311 = case shown="False" w700 {
                      tunnel: w699 -> [w701 w703]
                      tunnel: [w701 w702] -> w698
                      frame False {
                      }
                      frame True {
                        n312 = shared-variable "RT CompactRIO Target\\Mod4\\DO13"(TRUE ("DO15"), error in=w703) -> (error out=w702:errorcluster)
                      }
                    }
                  }
                  frame True {
                    n313 = shared-variable "RT CompactRIO Target\\Mod4\\DO12"(TRUE ("DO14"), error in=w706) -> (error out=w705:errorcluster)
                  }
                }
                n314 = Enqueue Element(queue=w695, element="MoveCenter", error in (no error)=w690) -> (queue out=w694:refnum<queue>, error out=w696:errorcluster)  [unwired: 1 in, 1 out]
              }
            }
          }
        }
      }
    }
    n315 = case shown="No Error" w496 {
      selector: w496 -> [w498 w502]
      tunnel: w495 -> [w499 w504]
      tunnel: [w499 w501] -> w494
      tunnel: [w498 w500] -> w492
      frame No Error {
      }
      frame Error {
        n316 = Enqueue Element(queue=w504, element="Shutdown") -> (queue out=w501:refnum<queue>, error out=w503:errorcluster)  [unwired: 2 in, 1 out]
        n317 = Merge Errors(w503, w502) -> (w500:errorcluster)
      }
    }
  }
  n318 = Release Queue(queue=w5) -> (error out=w3:errorcluster)  [unwired: 2 in, 2 out]
  n319 = Merge Errors(w3, w1) -> (→"error out":errorcluster)
